vi "Knob Fill Wrapper.vi"(8 "error in (no error)":errorcluster, 9 "Default Value Map":variant, 10 "Value":variant, 11 "Control Ref":refnum<vi>) -> ()   [LabVIEW 2019, in "User Interface.lvlib"]
doc: "Convenience wrapper for knob fill updates. Will accept and control ref type, and only perform updates if it's a knob control."
uses:
  User Interface.lvlib
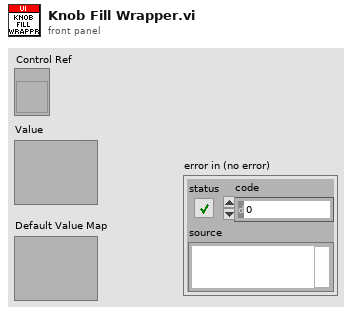
[diagram p1: front panel]
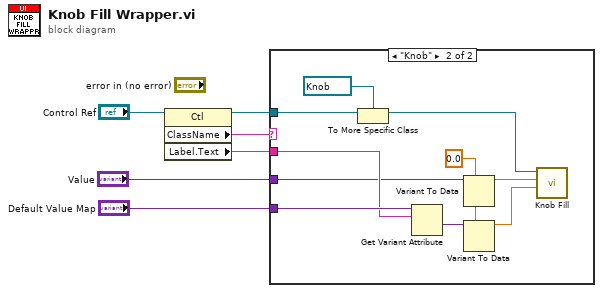
[diagram p0: block diagram]
diagram:
  n1 = property class="Ctl"(reference="Control Ref") -> (reference out=w5:refnum<vi>, "ClassName"=w4:string, "Label.Text"=w3:string)  [unwired: 1 in, 1 out]
  n2 = case shown="\"Knob\"" w4 {
    tunnel: w5 -> [_ w12]
    tunnel: w3 -> [_ w8]
    tunnel: "Default Value Map" -> [_ w9]
    tunnel: "Value" -> [_ w7]
    frame Default {
    }
    frame "Knob" {
      w14 = 0.0 ("y")
      n3 = To More Specific Class(target class=refnum<vi> refnum ("Knob Ref"), reference=w12) -> (specific class reference=w10:refnum<vi>)  [unwired: 1 in, 1 out]
      n4 = Get Variant Attribute(Variant=w9, name=w8) -> (value=w13:variant)  [unwired: 2 in, 3 out]
      n5 = Variant To Data(type=w14, Variant=w7) -> (data=w15:dbl)  [unwired: 1 in, 1 out]
      n6 = Variant To Data(type=w14, Variant=w13) -> (data=w16:dbl)  [unwired: 1 in, 1 out]
      n7 = call "Knob Fill.vi"("Default Value"=w16, "Value"=w15, "Knob Ref"=w10) -> ()  [unwired: 9 in]
    }
  }
